vi "Duplicate Name Error Test.vi"() -> (0 "error out":errorcluster, 1 "Success Error on Replace Line":bool, 2 "Success Error on Write Lines":bool, 3 "Success Error on Add":bool)   [LabVIEW 2015, in "UI Reference tests.lvlib"]
doc: "Tests the Add Line and Remove Line functions."
uses:
  UI Reference tests.lvlib
  <vilib>/NI/Tag Bus/tag/Data Type.ctl
  module/configuration/Line.ctl
  <vilib>/NI/Tag Bus Module Framework/channel/TBM channel.lvclass
  module/configuration/permissions.ctl
  module/configuration/Get Line Name.vi
  <vilib>/NI/Tag Bus Module Framework/module configuration/FindDuplicate.vi
  <vilib>/Utility/error.llb/Error Cluster From Error Code.vi
  module/configuration/UI Reference configuration.lvclass
  <vilib>/NI/Tag Bus/tag/tag descriptor.lvclass
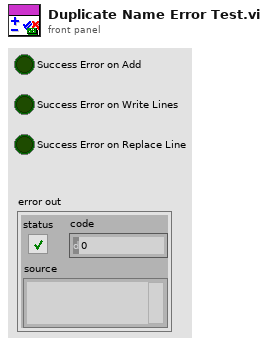
[diagram p1: front panel]
types:
  T1 = typedef "UI Reference configuration.lvclass/permissions.ctl" = enum32{"Read from Control", "Write to Indicator"}
  T2 = typedef "UI Reference configuration.lvclass/Line.ctl" = cluster{"channel":refnum<class "TBM channel.lvclass">}
  T3 = typedef "tag bus.lvlib/tag descriptor.lvclass/Data Type.ctl" = enum16{"Double", "Single", "I64", "I32", "I16", "I8", "U64", "U32", "U16", "U8", "Boolean", "String", "Array of Double", "Array of Single", "Array of I64", "Array of I32", "Array of I16", "Array of I8", "Array of U64", "Array of U32", "Array of U16", "Array of U8", "Array of Boolean", "Array of String"}
  T4 = typedef "TBM channel.lvclass/channel classification.ctl" = enum16{"input data", "output data", "processing parameter", "processing result"}
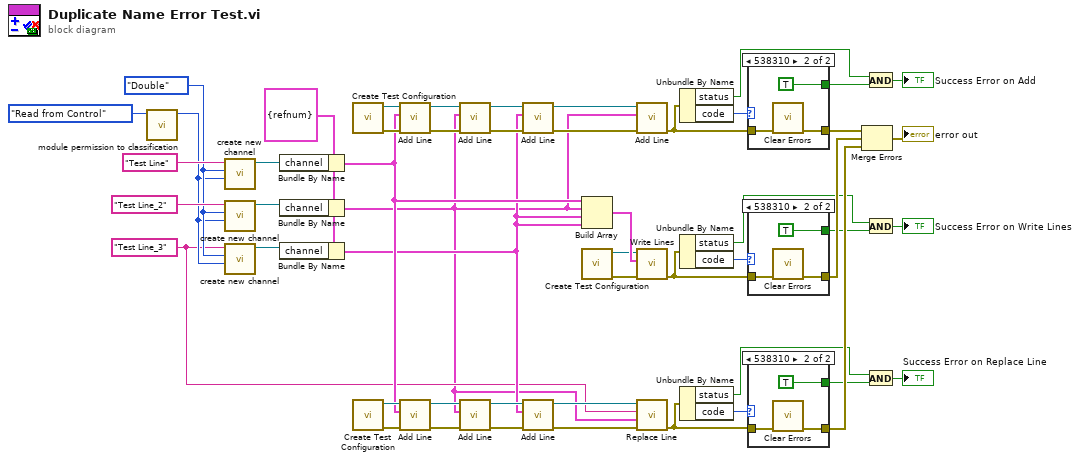
[diagram p0: block diagram]
diagram:
  w16 = "Test Line_3" ("channel name")
  w43 = T2 {"channel"=refnum} ("Line")
  w38 = Data_Type."Double" ("data type")
  n1 = call "module permission to classification.vi"("display permissions"=permissions."Read from Control") -> ("channel classification"=w37:T4)  [unwired: 10 in]
  n2 = call <vilib>:"create new channel.vi"("channel classification"=w37, "data type"=w38, "channel name"="Test Line") -> ("channel"=w50:refnum<class "TBM channel.lvclass">)  [unwired: 8 in]
  n3 = call <vilib>:"create new channel.vi"("channel classification"=w37, "data type"=w38, "channel name"="Test Line_2") -> ("channel"=w45:refnum<class "TBM channel.lvclass">)  [unwired: 8 in]
  n4 = call <vilib>:"create new channel.vi"("channel classification"=w37, "data type"=w38, "channel name"=w16) -> ("channel"=w44:refnum<class "TBM channel.lvclass">)  [unwired: 8 in]
  n5 = Bundle By Name(cluster=w43, "channel"=w50) -> (w19:T2)
  n6 = Bundle By Name(cluster=w43, "channel"=w45) -> (w15:T2)
  n7 = Bundle By Name(cluster=w43, "channel"=w44) -> (w18:T2)
  n8 = call "Create Test Configuration.vi"() -> ("error out"=w49:errorcluster, "Module Configuration"=w51:refnum<class "UI Reference configuration.lvclass">)  [unwired: 6 in, 4 out]
  n9 = call "Create Test Configuration.vi"() -> ("error out"=w21:errorcluster, "Module Configuration"=w20:refnum<class "UI Reference configuration.lvclass">)  [unwired: 6 in, 4 out]
  n10 = call "Add Line.vi"("error in"=w49, "Line"=w19, "UI Reference configuration in"=w51) -> ("error out"=w42:errorcluster, "UI Reference configuration out"=w39:refnum<class "UI Reference configuration.lvclass">)  [unwired: 6 in, 1 out]
  n11 = call "Add Line.vi"("error in"=w21, "Line"=w19, "UI Reference configuration in"=w20) -> ("error out"=w22:errorcluster, "UI Reference configuration out"=w25:refnum<class "UI Reference configuration.lvclass">)  [unwired: 6 in, 1 out]
  n12 = call "Add Line.vi"("error in"=w42, "Line"=w15, "UI Reference configuration in"=w39) -> ("error out"=w41:errorcluster, "UI Reference configuration out"=w40:refnum<class "UI Reference configuration.lvclass">)  [unwired: 6 in, 1 out]
  n13 = call "Add Line.vi"("error in"=w22, "Line"=w15, "UI Reference configuration in"=w25) -> ("error out"=w23:errorcluster, "UI Reference configuration out"=w24:refnum<class "UI Reference configuration.lvclass">)  [unwired: 6 in, 1 out]
  n14 = call "Add Line.vi"("error in"=w41, "Line"=w18, "UI Reference configuration in"=w40) -> ("error out"=w35:errorcluster, "UI Reference configuration out"=w36:refnum<class "UI Reference configuration.lvclass">)  [unwired: 6 in, 1 out]
  n15 = call "Add Line.vi"("error in"=w23, "Line"=w18, "UI Reference configuration in"=w24) -> ("error out"=w14:errorcluster, "UI Reference configuration out"=w17:refnum<class "UI Reference configuration.lvclass">)  [unwired: 6 in, 1 out]
  n16 = Build Array(w19, w15, w18, w18) -> (w32:T2[])
  n17 = call "Create Test Configuration.vi"() -> ("error out"=w13:errorcluster, "Module Configuration"=w31:refnum<class "UI Reference configuration.lvclass">)  [unwired: 6 in, 4 out]
  n18 = call "Add Line.vi"("error in"=w35, "Line"=w15, "UI Reference configuration in"=w36) -> ("error out"=w33:errorcluster)  [unwired: 6 in, 2 out]
  n19 = call "Write Lines.vi"("error in (no error)"=w13, "Lines"=w32, "UI Reference configuration in"=w31) -> ("error out"=w29:errorcluster)  [unwired: 7 in, 1 out]
  n20 = call "Replace Line.vi"("error in"=w14, "New Line"=w15, "Line Name"=w16, "UI Reference configuration in"=w17) -> ("error out"=w11:errorcluster)  [unwired: 5 in, 2 out]
  n21 = Unbundle By Name(w33) -> ("status"=w8:bool, "code"=w34:i32)
  n22 = Unbundle By Name(w29) -> ("status"=w3:bool, "code"=w30:i32)
  n23 = Unbundle By Name(w11) -> ("status"=w4:bool, "code"=w12:i32)
  n24 = case shown="538310" w34 {
    tunnel: w33 -> [w52 w55]
    tunnel: [w52 w54] -> w28
    tunnel: [_ TRUE ("Success Error on Add")] -> w9
    frame 0, Default {
    }
    frame 538310 {
      n25 = call <vilib>:"Clear Errors.vi"("error in (no error)"=w55) -> ("error out"=w54:errorcluster)  [unwired: 5 in, 1 out]
    }
  }
  n26 = case shown="538310" w30 {
    tunnel: w29 -> [w56 w59]
    tunnel: [w56 w58] -> w27
    tunnel: [_ TRUE ("Success Error on Add")] -> w2
    frame 0, Default {
    }
    frame 538310 {
      n27 = call <vilib>:"Clear Errors.vi"("error in (no error)"=w59) -> ("error out"=w58:errorcluster)  [unwired: 5 in, 1 out]
    }
  }
  n28 = case shown="538310" w12 {
    tunnel: w11 -> [w60 w63]
    tunnel: [w60 w62] -> w10
    tunnel: [_ TRUE ("Success Error on Add")] -> w5
    frame 0, Default {
    }
    frame 538310 {
      n29 = call <vilib>:"Clear Errors.vi"("error in (no error)"=w63) -> ("error out"=w62:errorcluster)  [unwired: 5 in, 1 out]
    }
  }
  n30 = Merge Errors(w28, w27, w10) -> (→"error out":errorcluster)
  n31 = And(x=w8, y=w9) -> (x .and. y?=→"Success Error on Add":bool)
  n32 = And(x=w3, y=w2) -> (x .and. y?=→"Success Error on Write Lines":bool)
  n33 = And(x=w4, y=w5) -> (x .and. y?=→"Success Error on Replace Line":bool)
